vi "www template process login keys.vi"(8 "error in (no error)":errorcluster, 11 "ENV":T1) -> (0 "error out":errorcluster, 3 "Login Keys":T1)   [LabVIEW 2011]
uses:
  ITK EXT/utils/keyedarr.llb/Keyed Array.ctl
  license/Authorization Global.vi
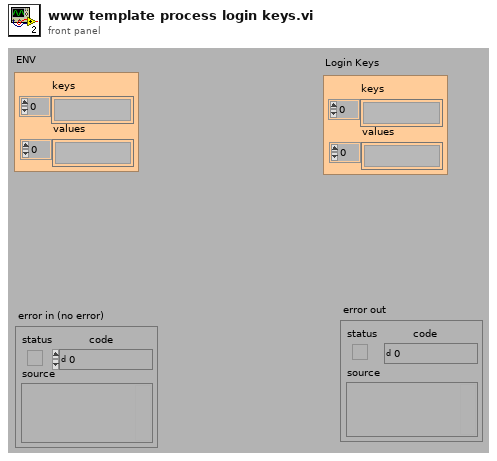
[diagram p1: front panel]
types:
  T1 = typedef "Keyed Array.ctl" = cluster{"keys":string[], "values":string[]}
  T2 = typedef "Authorization Data.ctl" = cluster{"Valid":bool, "Seats":i32, "Expire Time":timestamp, "Last Access Time":timestamp, "Product ID":string, "Hardware ID":string, "Spartan Serial Number":string, "Feature":cluster{"#attributes":cluster{"Name":string, "Value":string}}[]}
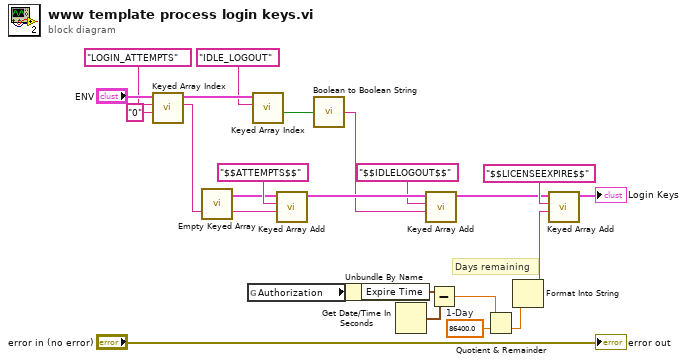
[diagram p0: block diagram]
diagram:
  w6 = 86400.0  # 1-Day
  # "Days remaining"
  n1 = call "Keyed Array Index.vi"("default value"="0", "key"="LOGIN_ATTEMPTS", "array in"="ENV") -> ("value"=w15:string, "duplicate array"=w14:T1)  [unwired: 1 in, 2 out]
  n2 = call "Empty Keyed Array.vi"() -> ("empty keyed array"=w19:T1)  [unwired: 3 out]
  n3 = global read "Authorization Global.vi" "Authorization"() -> (w2:T2)
  n4 = call "Keyed Array Index.vi"("key"="IDLE_LOGOUT", "array in"=w14) -> ("valid key"=w9:bool)  [unwired: 2 in, 3 out]
  n5 = call "Keyed Array Add.vi"("value"=w15, "key"="$$ATTEMPTS$$", "array in"=w19) -> ("array out"=w12:T1)  [unwired: 1 in, 3 out]
  n6 = call "Boolean to Boolean String.vi"("Boolean"=w9) -> ("Boolean string"=w8:string)  [unwired: 1 in]
  n7 = Unbundle By Name(w2) -> ("Expire Time"=w1:timestamp)
  n8 = Get Date/Time In Seconds() -> (seconds since 1Jan1904=w7:timestamp)
  n9 = call "Keyed Array Add.vi"("value"=w8, "key"="$$IDLELOGOUT$$", "array in"=w12) -> ("array out"=w11:T1)  [unwired: 1 in, 3 out]
  n10 = Subtract(x=w1, y=w7) -> (x-y=w5:dbl)
  n11 = Quotient & Remainder(x=w5, y=w6) -> (floor(x/y)=w4:dbl)  [unwired: 1 out]
  n12 = Format Into String(w4) -> (resulting string=w23:string)  [unwired: 3 in, 1 out]
  n13 = call "Keyed Array Add.vi"("value"=w23, "key"="$$LICENSEEXPIRE$$", "array in"=w11) -> ("array out"=→"Login Keys":T1)  [unwired: 1 in, 3 out]
  "error out" <- "error in (no error)"
